vi "GetPower.vi"(8 "error in (no error)":errorcluster, 10 "Label":string, 11 "Laser_Oxxius in":refnum<class "Laser_Oxxius.lvclass">) -> (0 "error out":errorcluster, 2 "Value":dbl format="%#_13g", 3 "Laser_Oxxius out":refnum<class "Laser_Oxxius.lvclass">)   [LabVIEW 2020, in "Laser_Oxxius.lvlib" / "Laser_Oxxius.lvclass"]
uses:
  Laser_Oxxius.lvclass
  Laser_Oxxius.lvclass/Laser_Oxxius.ctl
  E:/Development/DevHardSoftware/MicroscopyFramework/Model/Hardware Layer/Real Hardware/Laser_Oxxius/Laser_Oxxius/Dependency/Oxxius_Boxx.dll
  Dependency/Oxxius_Boxx.dll
  Hardware Abstraction Layer/Component/Laser/Laser/Laser.lvclass
panel:
  in  "event data":cluster{"Label":string, "Value":dbl}
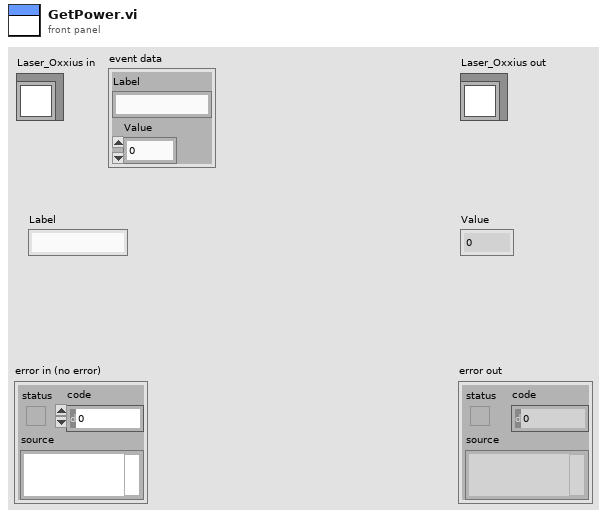
[diagram p1: front panel]
types:
  T1 = typedef "DataListener.lvclass/DataExchange.ctl" = cluster{"Source":string, "Destination":string, "Description":string, "value":variant}
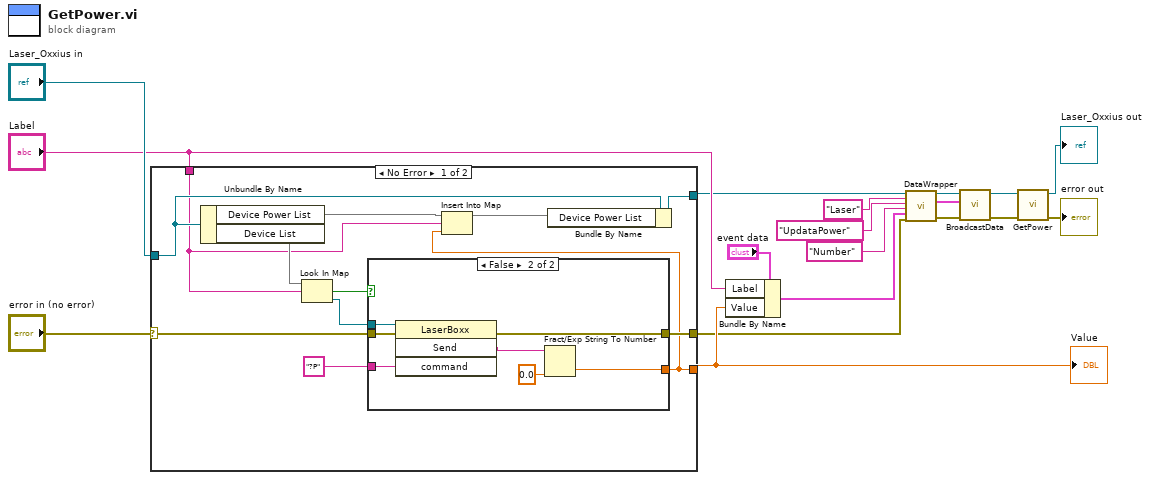
[diagram p0: block diagram]
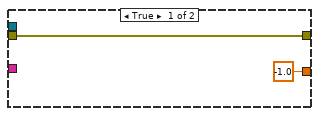
[diagram p2: hidden frame]
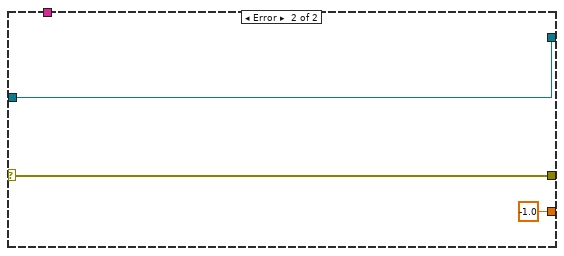
[diagram p3: hidden frame]
diagram:
  n1 = case shown="No Error" "error in (no error)" {
    selector: "error in (no error)" -> [w30 w42]
    tunnel: "Laser_Oxxius in" -> [w24 w40]
    tunnel: [w27 w42] -> w6
    tunnel: "Label" -> [w20 _]
    tunnel: [w19 -1.0] -> w12
    tunnel: [w23 w40] -> w1
    frame No Error {
      n2 = Unbundle By Name(w24) -> ("Device Power List"=w22:map{string, dbl}, "Device List"=w29:map{string, refnum<k24>})
      n3 = Look In Map(map=w29, key=w20) -> (key not found?=w26:bool, value=w28:refnum<k24>)  [unwired: 1 in]
      n4 = case shown="False" w26 {
        tunnel: w30 -> [w32 w39]
        tunnel: w28 -> [_ w38]
        tunnel: [w32 w37] -> w27
        tunnel: "?P" ("command") -> [_ w36]
        tunnel: [-1.0 w33] -> w19
        frame True {
        }
        frame False {
          n5 = invoke class="LaserBoxx" method="Send"(reference=w38, error in=w39, "command"=w36) -> (error out=w37:errorcluster, "Send"=w34:string)  [unwired: 1 in, 2 out]
          n6 = Fract/Exp String To Number(string=w34, default (0 dbl)=0.0 ("default (0 DBL)")) -> (number=w33:dbl)  [unwired: 2 in, 1 out]
        }
      }
      n7 = Insert Into Map(map in=w22, key=w20, value=w19) -> (map out=w21:map{string, dbl})  [unwired: 2 out]
      n8 = Bundle By Name(cluster=w24, "Device Power List"=w21) -> (w23:refnum<class "Laser_Oxxius.lvclass">)
    }
    frame Error {
    }
  }
  "Value" <- w12
  n9 = Bundle By Name(cluster="event data", "Label"="Label", "Value"=w12) -> (w7:cluster{"Label":string, "Value":dbl})
  n10 = call-dynamic "DataWrapper.vi"("Device in"=w1, "Source"="Laser", "Description"="UpdataPower" ("Target"), "Destination"="Number" ("Type"), "value"=w7, "error in (no error)"=w6) -> ("Device out"=w11:refnum<class "Laser_Oxxius.lvclass">, "DataExchange"=w4:T1, "error out"=w3:errorcluster)  [unwired: 11 in]
  n11 = call-dynamic "BroadcastData.vi"("error in (no error)"=w3, "DataExchange"=w4, "Device in"=w11) -> ("error out"=w2:errorcluster, "Device out"=w5:refnum<class "Laser_Oxxius.lvclass">)  [unwired: 7 in]
  n12 = call-parent "GetPower.vi"("error in (no error)"=w2, "Laser in"=w5) -> ("error out"=→"error out":errorcluster, "Laser out"=→"Laser_Oxxius out":refnum<class "Laser_Oxxius.lvclass">)  [unwired: 7 in, 1 out]
